vi "Parameter Set Read Array.vi"(8 "error in (no error)":errorcluster, 11 "Parameter Set in":refnum<class "Parameter Set.lvclass">) -> (0 "error out":errorcluster, 1 "Changed or First Call?":bool, 2 "Parameter Set CTL":i32[](array[numeric]), 3 "Parameter Set out":refnum<class "Parameter Set.lvclass">)   [LabVIEW 2023, in "Parameter Set.lvclass"]
uses:
  Parameter Set.lvclass
  Parameter Set.lvclass/Parameter Set.ctl
  <vilib>/ADAS Replay HIL/Channels/Tag Wrapper/Polymorphic/Read Channel (I32).vi
  db239f6a-af45-49a9-94f3-89caea2bcc83.vi
  <vilib>/ADAS Replay HIL/Channels/Tag Wrapper/Polymorphic/Read Channel (I32).vi/b2f764de-0c1e-4784-a155-687fc995a684.vi
  <vilib>/ADAS Replay HIL/Channels/Tag Wrapper/Polymorphic/Read Channel (I32).vi/b2f764de-0c1e-4784-a155-687fc995a684.vi/c28b0ead-42ad-4072-80a2-aca7f2bd7ce3.vi
  <vilib>/ADAS Replay HIL/Channels/Tag Wrapper/Polymorphic/Read Channel (I32).vi/b2f764de-0c1e-4784-a155-687fc995a684.vi/219d0231-d98b-4193-b5cc-84f90e3c9091.vi
  <vilib>/ADAS Replay HIL/Channels/Tag Wrapper/Tag Wrapper.lvlib
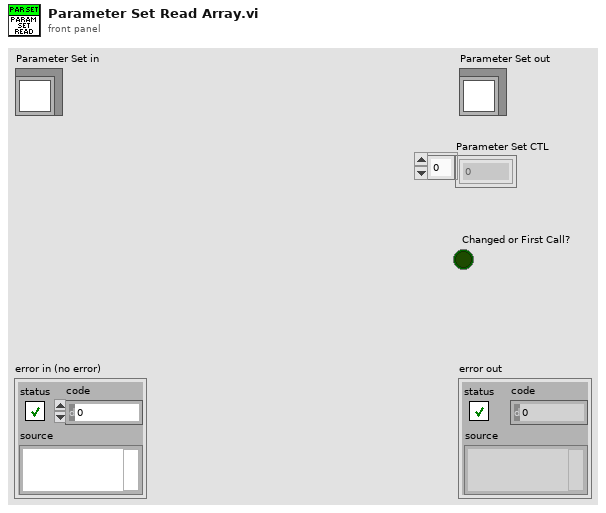
[diagram p1: front panel]
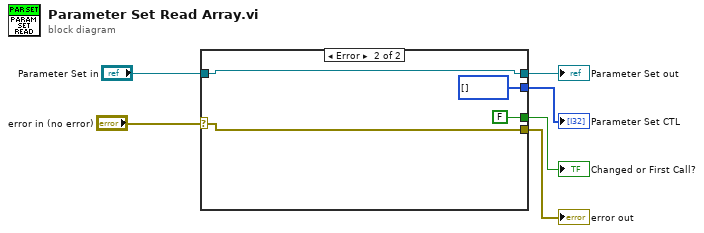
[diagram p0: block diagram]
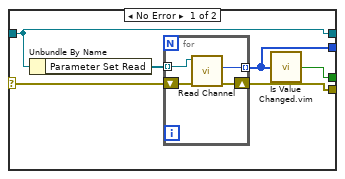
[diagram p2: hidden frame]
diagram:
  n1 = case shown="Error" "error in (no error)" {
    selector: "error in (no error)" -> [w10 w20]
    tunnel: [w9 w20] -> w5
    tunnel: [w11 w19] -> w3
    tunnel: "Parameter Set in" -> [w11 w19]
    tunnel: [w8 FALSE ("changed or first call?")] -> w2
    tunnel: [w7 i32[] []] -> w1
    frame No Error {
      n2 = Unbundle By Name(w11) -> ("Parameter Set Read"=w12:refnum<k21>[])
      n3 = for {
        tunnel: [w14] -> w7 mode=indexing
        shift-right: [w15] -> w9
        shift-left: w10 -> [w16]
        tunnel: w12 -> [w13] mode=indexing
        n4 = call-poly <vilib>:"Read Channel.vi"("error in"=w16, "ADAS HIL Channel in"=w13) -> ("error out"=w15:errorcluster, "Value out"=w14:i32)  [unwired: 6 in, 2 out]
      }
      n5 = call "Is Value Changed.vim"("value"=w7) -> ("changed or first call?"=w8:bool)
    }
    frame Error {
    }
  }
  "error out" <- w5
  "Parameter Set out" <- w3
  "Parameter Set CTL" <- w1
  "Changed or First Call?" <- w2
